vi "Init.vi"(8 "Error In":errorcluster, 10 "Folder Path":path, 11 "Plugin Framework In":refnum<class "Factory Plugin Framework.lvclass">=refnum) -> (0 "Error Out":errorcluster, 3 "Factory Plugin Framework out":refnum<class "Factory Plugin Framework.lvclass">)   [LabVIEW 2018, in "Factory Plugin Framework.lvlib" / "Factory Plugin Framework.lvclass"]
uses:
  Factory Plugin Framework.lvclass
  Factory Plugin Framework.lvclass/Factory Plugin Framework.ctl
  Accessors/Write Plugin Type.vi
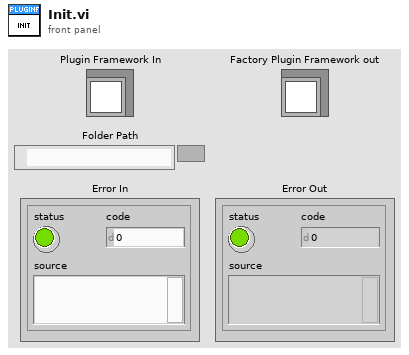
[diagram p1: front panel]
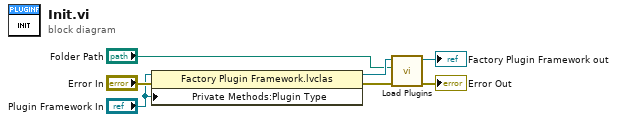
[diagram p0: block diagram]
diagram:
  n1 = property class="Factory Plugin Framework.lvclas"(reference="Plugin Framework In", error in="Error In", "Private Methods:Plugin Type"="Plugin Framework In") -> (reference out=w7:refnum<class "Factory Plugin Framework.lvclass">, error out=w6:errorcluster)
  n2 = call "Load Plugins.vi"("Error In"=w6, "Folder Path"="Folder Path", "Factory Plugin Framework in"=w7) -> ("Error Out"=→"Error Out":errorcluster, "Factory Plugin Framework out"=→"Factory Plugin Framework out":refnum<class "Factory Plugin Framework.lvclass">)  [unwired: 7 in]
